vi "Read Event Log Credentials.vi"(11 "IMediator in":refnum<class "IMediator.lvclass">) -> (1 "Framework Instance Alias":string, 2 "Event Log Instance":refnum<class "LoggerReference.lvclass">)   [LabVIEW 2017, in "IMediator.lvlib" / "IMediator.lvclass"]
uses:
  IMediator.lvclass
  gpm_packages/@cs/event-logger/Source/Composed Log/LoggerReference/LoggerReference.lvclass
  IMediator.lvclass/IMediator.ctl
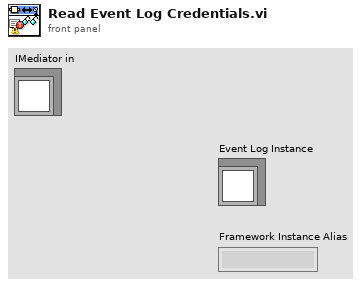
[diagram p1: front panel]
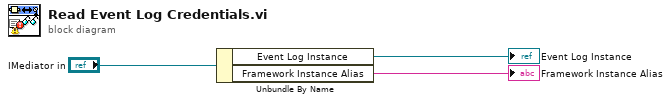
[diagram p0: block diagram]
diagram:
  n1 = Unbundle By Name("IMediator in") -> ("Event Log Instance"=→"Event Log Instance":refnum<class "LoggerReference.lvclass">, "Framework Instance Alias"=→"Framework Instance Alias":string)
